vi "Dispose LCOS Images.vi"(0 "Images":T1) -> ()   [LabVIEW 2011]
uses:
  LCOS Images.ctl
  <vilib>/vision/Image Controls.llb/IMAQ Image.ctl
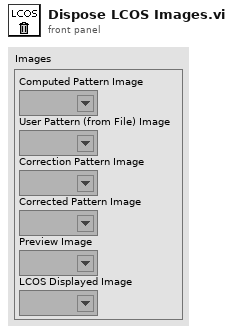
[diagram p1: front panel]
types:
  T1 = typedef "LCOS Images.ctl" = cluster{"Computed Pattern Image":T2, "User Pattern (from File) Image":T2, "Correction Pattern Image":T2, "Corrected Pattern Image":T2, "Preview Image":T2, "LCOS Displayed Image":T2}
  T2 = typedef "IMAQ Image.ctl" = refnum<image>
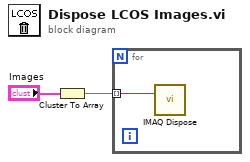
[diagram p0: block diagram]
diagram:
  n1 = Cluster To Array(cluster="Images") -> (array=w1:T2[])
  n2 = for {
    tunnel: w1 -> [w3] mode=indexing
    n3 = call "IMAQ Dispose"("Image"=w3) -> ()  [unwired: 5 in, 1 out]
  }
